vi "Pearson’s R.vi"(8 "1D":dbl[](array[numeric]) format="%#_2g", 11 "2D":i32[][](array[numeric])) -> (0 "kpC Chart":dbl[](graph), 3 "kpC":dbl[](array[numeric]) format="%#_3g")   [LabVIEW 2023]
panel:
  out "std[i]":dbl
  out "std 1":dbl[](array[numeric]) format="%#_4g"
  out "std 2":dbl[](array[numeric]) format="%#_4g"
  out "El CNT":i32
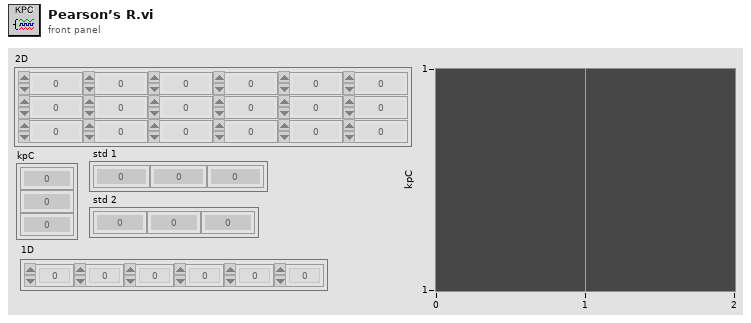
[diagram p1: front panel]
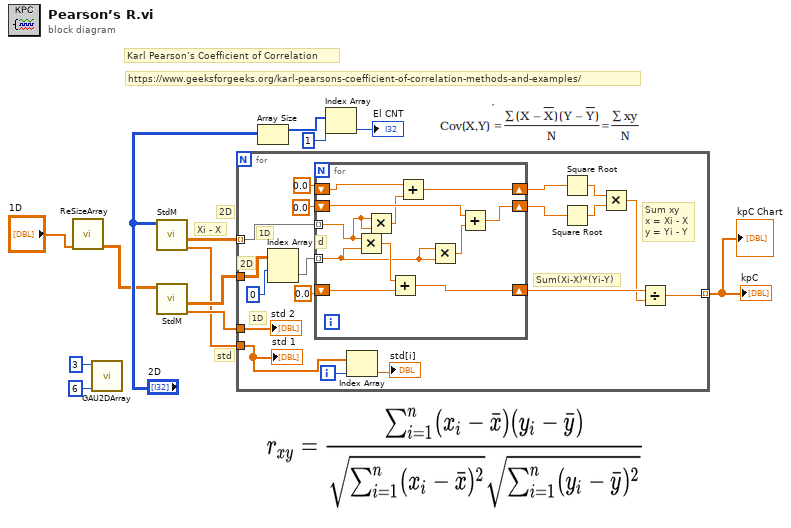
[diagram p0: block diagram]
diagram:
  # "https://www.geeksforgeeks.org/karl-pearsons-coefficient-of-correlation-methods-and-examples/"
  # "Karl Pearson’s Coefficient of Correlation"
  # "std"
  # "Xi - X"
  # "2D"
  n1 = call "ReSizeArray.vi"("Array"="1D") -> ("1D to 2D"=w1:dbl[][])  [unwired: 9 in, 1 out]
  n2 = call "GAU2DArray.vi"("Colums"=6, "Rows"=3) -> ()  [unwired: 7 in, 3 out]
  n3 = call "StdM.vi"("2D"="2D") -> ("My std"=w4:dbl[], "[Xi-X]"=w7:dbl[][])  [unwired: 6 in, 3 out]
  n4 = call "StdM.vi"("2D"=w1) -> ("My std"=w5:dbl[], "[Xi-X]"=w6:dbl[][])  [unwired: 6 in, 3 out]
  n5 = for {
    tunnel: w7 -> [w31] mode=indexing
    tunnel: w6 -> [w27]
    tunnel: w5 -> [w30]
    tunnel: w4 -> [w29]
    tunnel: [w21] -> w3 mode=indexing
    i -> [w22]
    # "Sum xy\nx = Xi - X\ny = Yi - Y"
    # "Sum(Xi-X)*(Yi-Y)"
    # "2D"
    # "1D"
    # "1D"
    n6 = Index Array(array=w27, index (row)=0) -> (element=w25:dbl[])  [unwired: 1 in]
    n7 = for {
      tunnel: w31 -> [w35] mode=indexing
      tunnel: w25 -> [w33] mode=indexing
      shift-right: [w41] -> w24
      shift-left: 0.0 -> [w40]
      shift-right: [w39] -> w18
      shift-left: 0.0 -> [w36]
      shift-right: [w38] -> w17
      shift-left: 0.0 -> [w37]
      # "d"
      n8 = Multiply(x=w35, y=w33) -> (x*y=w42:dbl)
      n9 = Multiply(x=w35, y=w35) -> (x*y=w34:dbl)
      n10 = Add(x=w42, y=w40) -> (x+y=w41:dbl)
      n11 = Add(x=w36, y=w34) -> (x+y=w39:dbl)
      n12 = Multiply(x=w33, y=w33) -> (x*y=w32:dbl)
      n13 = Add(x=w37, y=w32) -> (x+y=w38:dbl)
    }
    n14 = Index Array(array=w29, index=w22) -> (element=→"std[i]":dbl)
    n15 = Square Root(x=w18) -> (sqrt(x)=w15:dbl)
    n16 = Square Root(x=w17) -> (sqrt(x)=w16:dbl)
    n17 = Multiply(x=w15, y=w16) -> (x*y=w14:dbl)
    n18 = Divide(x=w24, y=w14) -> (x/y=w21:dbl)
    "std 2" <- w30
    "std 1" <- w29
  }
  "kpC Chart" <- w3
  "kpC" <- w3
  n19 = Array Size(array="2D") -> (size(s)=w13:i32[])
  n20 = Index Array(array=w13, index=1) -> (element=→"El CNT":i32)
